vi "Analyze all images in GEECS tdms file.vi"(8 "error in (no error)":errorcluster, 11 "file path":path) -> (0 "error out":errorcluster, 3 "Intensity Graph":u16[][](graph))   [LabVIEW 2020]
uses:
  <userlib>/_MGI/File/Spreadsheet/MGI Write Spreadsheet Behavior Enum.ctl
panel:
  out "property value":string
  out "group/channel names":string[][](array[string])
  out "channel name":string
  out "group names":string[](array[string])
  out "image # -1":i32
  in  "stop":bool
  out "# pix per image":i32
  out "found":bool
  out "width":i32
  out "size(s)":i32
  out "time to read":u32
  out "data":u16[](array[numeric])
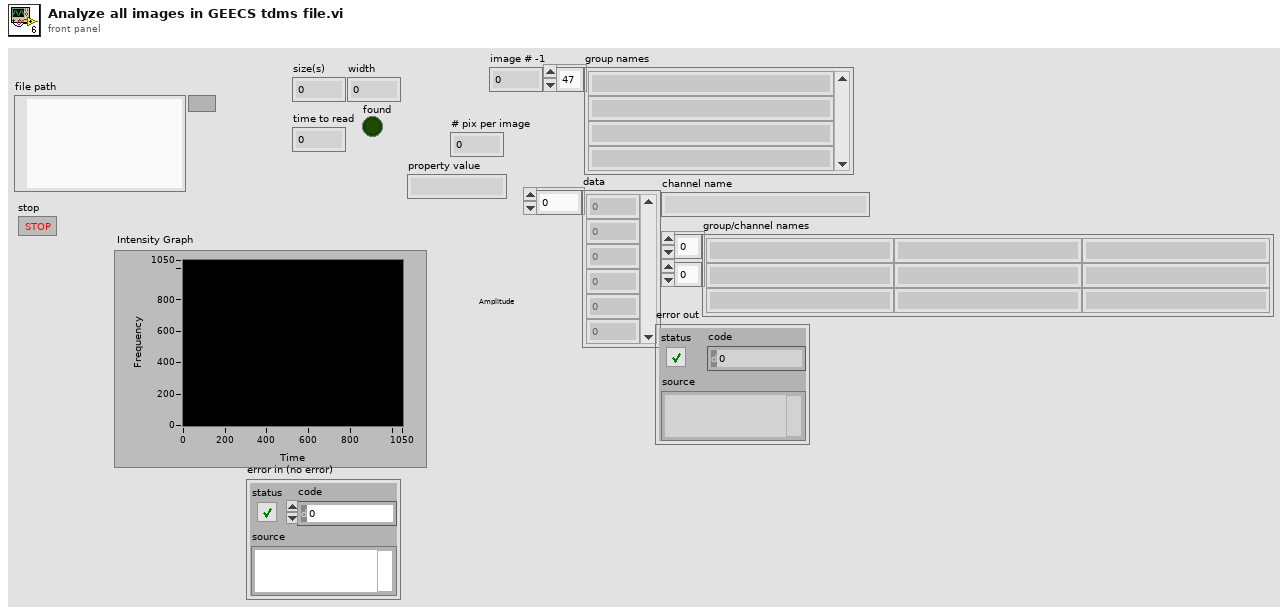
[diagram p1: front panel]
types:
  T1 = enum16{"open", "open or create", "create or replace", "create", "open (read-only)"}
  T2 = typedef "Image Type" = u32
  T3 = typedef "IMAQ Image.ctl" = refnum<image>
  T4 = typedef "MGI Write Spreadsheet Behavior Enum.ctl" = enum16{"Append data", "Append headers and data", "Overwrite"}
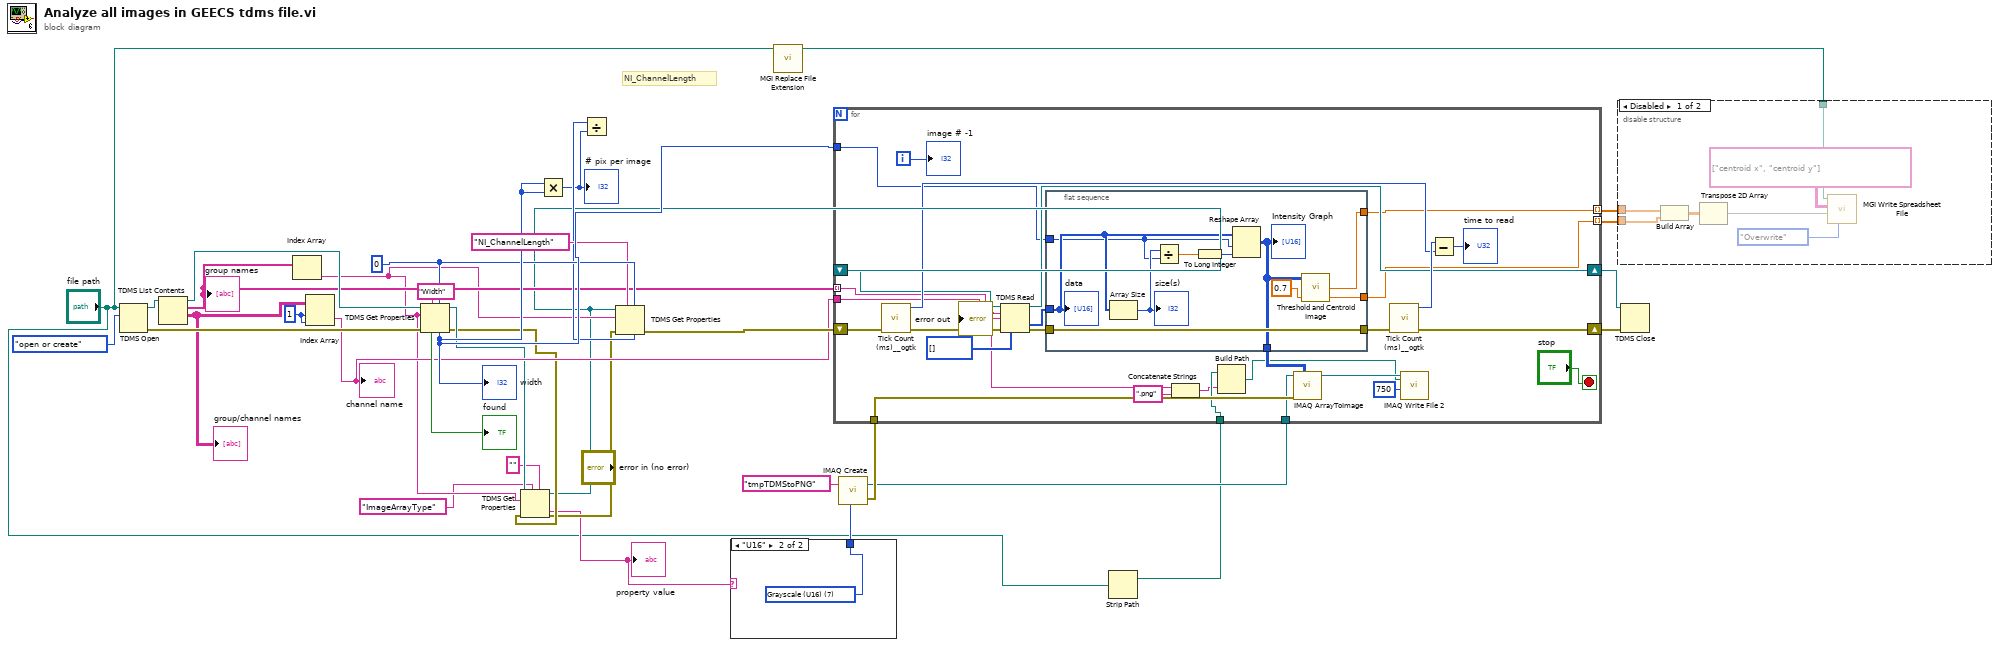
[diagram p0: block diagram]
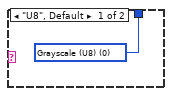
[diagram p3: hidden frame]
diagram:
  w18 = 1 ("index (row)")
  w29 = 0 ("x")
  # "NI_ChannelLength"
  n1 = TDMS Open(10:T1."open or create" ("operation (0:open)"), 11:"file path") -> (0:w33:errorcluster, 3:w20:refnum<k34>)  [unwired: 5 in]
  n2 = TDMS List Contents(7:w20) -> (1:w19:string[][], 2:w15:string[], 3:w17:refnum<k34>)  [unwired: 2 in, 1 out]
  "group names" <- w15
  "group/channel names" <- w19
  n3 = Index Array(array=w15) -> (element=w14:string)  [unwired: 1 in]
  n4 = Index Array(array=w19, index (row)=w18, index (col)=w18) -> (element=w16:string)
  "channel name" <- w16
  n5 = TDMS Get Properties(5:w29, 7:"Width", 8:w33, 10:w14, 11:w17) -> (0:w11:errorcluster, 3:w13:refnum<k34>, 4:w30:i32, 6:→"found":bool)  [unwired: 1 in, 2 out]
  "width" <- w30
  n6 = TDMS Get Properties(5:"" ("data type"), 7:"ImageArrayType", 8:w11, 10:w14, 11:w13) -> (0:w10:errorcluster, 3:w9:refnum<k34>, 4:w7:string)  [unwired: 1 in, 3 out]
  "property value" <- w7
  n7 = Multiply(x=w30, y=w30) -> (x*y=w26:i32)
  "# pix per image" <- w26
  n8 = TDMS Get Properties(5:w29, 7:"NI_ChannelLength" ("property name"), 8:w10, 10:w14, 11:w9) -> (0:w25:errorcluster, 4:w27:i32)  [unwired: 1 in, 4 out]
  n9 = Divide(x=w27, y=w26) -> ()  [unwired: 1 out]
  n10 = case shown="\"U16\"" w7 {
    tunnel: [w36 w37] -> w6
    frame "U8", Default {
      w36 = T2 0 items=["Grayscale (U8)", "Grayscale (I16)", "Grayscale (SGL)", "Complex (CSG)", "RGB (U32)", "HSL (U32)", "RGB (U64)", "Grayscale (U16)"] ("Image Type")
    }
    frame "U16" {
      w37 = T2 7 items=["Grayscale (U8)", "Grayscale (I16)", "Grayscale (SGL)", "Complex (CSG)", "RGB (U32)", "HSL (U32)", "RGB (U64)", "Grayscale (U16)"] ("Image Type")
    }
  }
  n11 = call <userlib>:"MGI Replace File Extension.vi"("Path In"="file path") -> ("Path Out"=w21:path)  [unwired: 9 in, 1 out]
  n12 = call "IMAQ Create"("Image Name"="tmpTDMStoPNG", "Image Type"=w6) -> ("New Image"=w3:T3, "error out"=w4:errorcluster)  [unwired: 3 in]
  n13 = Strip Path(path="file path") -> (stripped path=w1:path)  [unwired: 1 out]
  n14 = for {
    tunnel: w30 -> [w57]
    tunnel: w15 -> [w41] mode=indexing
    tunnel: w16 -> [w56]
    shift-right: [w61] -> w34
    shift-left: w9 -> [w54]
    shift-right: [w52] -> w24
    shift-left: w25 -> [w53]
    tunnel: [w49] -> w23 mode=indexing
    tunnel: [w48] -> w22 mode=indexing
    tunnel: w4 -> [w46]
    tunnel: w3 -> [w45]
    tunnel: w1 -> [w42]
    i -> [w50]
    stop <- "stop" stop-if-true
    n15 = call <userlib>:"Tick Count (ms)__ogtk.vi"("error in (no error)"=w53) -> ("error out"=w64:errorcluster, "millisecond timer value"=w62:u32)  [unwired: 9 in]
    n16 = TDMS Read(0:w54, 5:w41, 7:w56, 11:w64, 12:u16[] [] ("output array")) -> (4:w61:refnum<k34>, 10:w59:u16[], 15:w55:errorcluster)  [unwired: 3 in, 3 out]
    n17 = flat-sequence {
      tunnel: w59 -> [w75]
      tunnel: w57 -> [w71]
      tunnel: w55 -> [w70]
      tunnel: [w70] -> w58
      tunnel: [w68] -> w49
      tunnel: [w67] -> w48
      tunnel: [w66] -> w43
      frame #0 {
        n18 = Array Size(array=w75) -> (size(s)=w74:i32)
        "size(s)" <- w74
        n19 = Divide(x=w74, y=w71) -> (x/y=w73:dbl)
        n20 = To Long Integer(number=w73) -> (32bit integer=w72:i32)
        n21 = Reshape Array(w75, w71, w72) -> (w66:u16[][])
        "Intensity Graph" <- w66
        n22 = call "Threshold and Centroid Image.vi"("Raw Image"=w66, "Threshold or Threshold Fraction*"=0.7) -> ("x0"=w68:dbl, "y0"=w67:dbl)  [unwired: 2 in, 4 out]
        "data" <- w75
      }
    }
    n23 = Concatenate Strings(w41, ".png" ("string")) -> (w40:string)
    n24 = Build Path(base path=w42, name or relative path=w40) -> (appended path=w38:path)
    n25 = call "IMAQ ArrayToImage"("Image Pixels (U16)"=w43, "error in (no error)"=w46, "Image"=w45) -> ("Image Out"=w47:T3)  [unwired: 7 in, 1 out]
    n26 = call <userlib>:"Tick Count (ms)__ogtk.vi"("error in (no error)"=w58) -> ("error out"=w52:errorcluster, "millisecond timer value"=w63:u32)  [unwired: 9 in]
    n27 = call-poly "IMAQ Write File 2"("Image Quality"=u32 750, "File Path"=w38, "Image"=w47) -> ()  [unwired: 7 in, 2 out]
    n28 = Subtract(x=w63, y=w62) -> (x-y=→"time to read":u32)
    "image # -1" <- w50
  }
  n29 = disable-structure shown="Disabled" {
    disable-tunnel: w23 -> [w82 _]
    disable-tunnel: w22 -> [w81 _]
    disable-tunnel: w21 -> [w78 _]
    frame Disabled {
      n30 = Build Array(w82, w81) -> (w80:dbl[][])
      n31 = Transpose 2D Array(2D array=w80) -> (transposed array=w76:dbl[][])
      n32 = call <userlib>:"MGI Write Spreadsheet File.vi"("Existing File Behavior"=MGI_Write_Spreadsheet_Behavior_Enum."Overwrite", "Data[row][col]"=w76, "Header Lines[row][col]"=string[][] [["centroid x", "centroid y"]], "Path"=w78) -> ()  [unwired: 4 in, 4 out]
    }
    frame Enabled {
    }
  }
  n33 = TDMS Close(8:w24, 11:w34) -> ()  [unwired: 2 out]
